vi "basic_oe.vi"() -> ()   [LabVIEW 2017]
panel:
  out "Boolean":bool
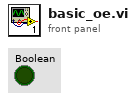
[diagram p1: front panel]
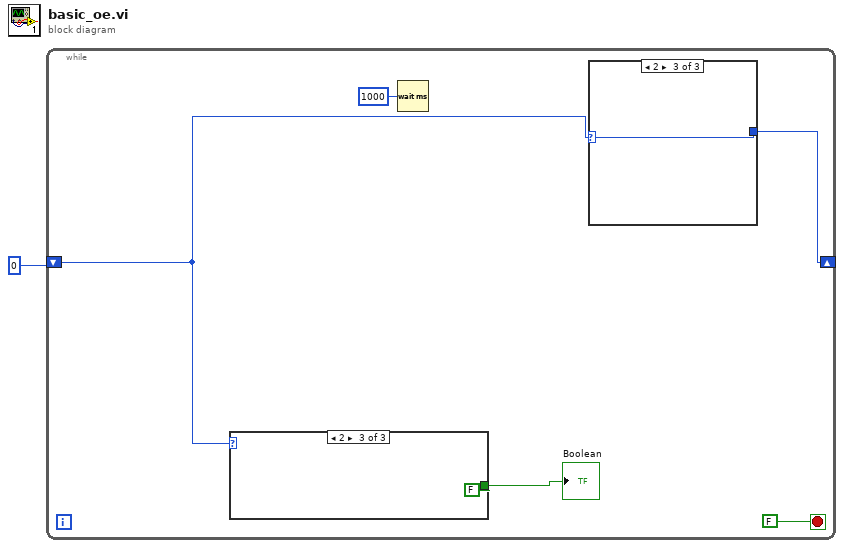
[diagram p0: block diagram]
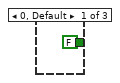
[diagram p2: hidden frame]
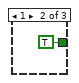
[diagram p3: hidden frame]
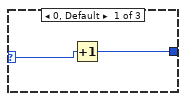
[diagram p4: hidden frame]
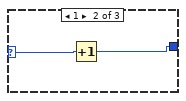
[diagram p5: hidden frame]
diagram:
  n1 = while {
    shift-right: [w5] -> _
    shift-left: 0 -> [w3]
    stop <- FALSE stop-if-true
    n2 = case shown="2" w3 {
      tunnel: [FALSE TRUE FALSE] -> w2
      frame 0, Default {
      }
      frame 1 {
      }
      frame 2 {
      }
    }
    "Boolean" <- w2
    n3 = Wait (ms)(milliseconds to wait=u32 1000) -> ()  [unwired: 1 out]
    n4 = case shown="2" w3 {
      selector: w3 -> [w11 w13 w14]
      tunnel: [w10 w12 w14] -> w5
      frame 0, Default {
        n5 = Increment(x=w11) -> (x+1=w10:i32)
      }
      frame 1 {
        n6 = Increment(x=w13) -> (x+1=w12:i32)
      }
      frame 2 {
      }
    }
  }
